vi "Cookies.vi"(11 "ID cookie":string) -> (3 "cookie header":string)   [LabVIEW 2014]
doc: "Prepares the cookie id and value and the Max-Age directive for the Set-Cookie header"
uses:
  Configuration/Global_Configurations.vi
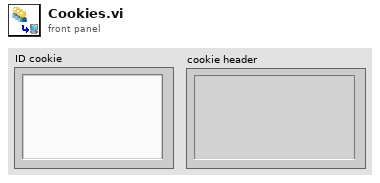
[diagram p1: front panel]
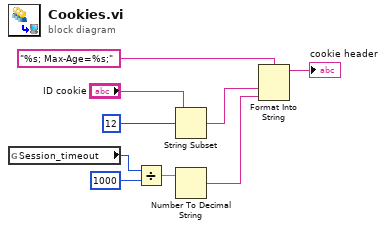
[diagram p0: block diagram]
diagram:
  n1 = global read "Global_Configurations.vi" "Session_timeout"() -> (w3:u32)
  n2 = Divide(x=w3, y=u32 1000) -> (x/y=w2:dbl)
  n3 = String Subset(string="ID cookie", offset (0)=12) -> (substring=w5:string)  [unwired: 1 in]
  n4 = Number To Decimal String(number=w2) -> (decimal integer string=w4:string)  [unwired: 1 in]
  n5 = Format Into String(format string="%s; Max-Age=%s;" ("string"), w5, w4) -> (resulting string=→"cookie header":string)  [unwired: 2 in, 1 out]
